vi "serialization tests.vi"() -> ()   [LabVIEW 2013, in "Profibus Module tests.lvlib"]
uses:
  Profibus Module tests.lvlib
  configuration/Profibus Module configuration.lvclass
panel:
  out "modules OK":bool
  out "no error":errorcluster
  out "no error":errorcluster
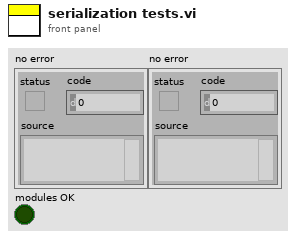
[diagram p1: front panel]
types:
  T1 = typedef "Profibus Module configuration.lvclass/endianness setting.ctl" = cluster{"slave":i8, "big endian":bool}
  T2 = typedef "Profibus Module configuration.lvclass/slave diagnostic configuration.ctl" = cluster{"slave":i8, "report":bool, "channel":refnum<class "TBM channel.lvclass">, "error specs":T3[]}
  T3 = typedef "Profibus Module configuration.lvclass/error throw specification.ctl" = cluster{"byte":i32, "bit":i32, "inverted?":bool, "error":i32}
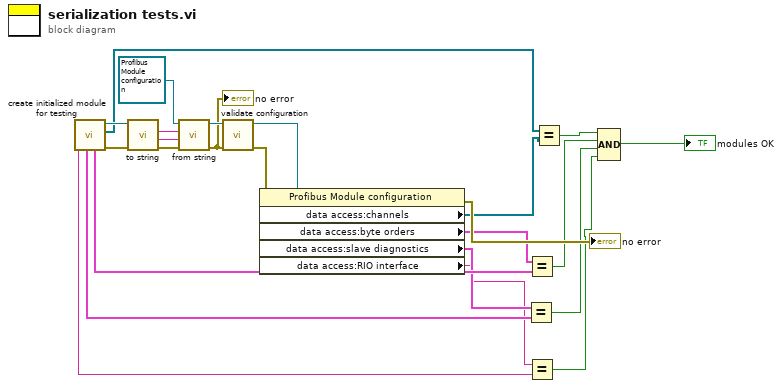
[diagram p0: block diagram]
diagram:
  n1 = call "create initialized module for testing.vi"() -> ("error out"=w16:errorcluster, "1d channels"=w11:refnum<class "Profibus channel.lvclass">[], "Profibus Module configuration out"=w17:refnum<class "Profibus Module configuration.lvclass">, "byte orders"=w7:T1[], "slave diagnostics"=w6:T2[], "RIO interface"=w2:string)  [unwired: 3 in, 3 out]
  n2 = call-dynamic "to string.vi"("error in"=w16, "Profibus Module configuration in"=w17) -> ("error out"=w24:errorcluster, "data"=w23:string, "version"=w22:string)  [unwired: 6 in, 1 out]
  n3 = call-dynamic "from string.vi"("error in"=w24, "data"=w23, "version"=w22, "Profibus Module configuration in"=refnum<class "Profibus Module configuration.lvclass"> refnum ("tag bus configurable plugin module configuration")) -> ("error out"=w20:errorcluster, "Profibus Module configuration out"=w21:refnum<class "Profibus Module configuration.lvclass">)  [unwired: 6 in]
  "no error" <- w20
  n4 = call-dynamic "validate configuration.vi"("error in"=w20, "Profibus Module configuration in"=w21) -> ("error out"=w15:errorcluster, "Profibus Module configuration out"=w14:refnum<class "Profibus Module configuration.lvclass">)  [unwired: 8 in]
  n5 = property class="Profibus Module configuration"(reference=w14, error in=w15) -> (error out=→"no error":errorcluster, "data access:channels"=w10:refnum<class "Profibus channel.lvclass">[], "data access:byte orders"=w4:T1[], "data access:slave diagnostics"=w5:T2[], "data access:RIO interface"=w3:string)  [unwired: 1 out]
  n6 = Equal?(x=w5, y=w6) -> (x = y?=w8:bool)
  n7 = Equal?(x=w4, y=w7) -> (x = y?=w9:bool)
  n8 = Equal?(x=w3, y=w2) -> (x = y?=w1:bool)
  n9 = Equal?(x=w11, y=w10) -> (x = y?=w19:bool)
  n10 = Compound Arithmetic op=AND(w19, w9, w8, w1) -> (→"modules OK":bool)
